vi "DO Block Config Pane.vi"(6 "_SubPanelMessages":refnum<notifier>, 9 "_myEmbeddedToFrameEvent":T7, 10 "_myEmbedded.Exit":refnum<user-event>, 11 "-Property Bundle":cluster{"Name":string, "Value":variant}[](array[cluster])) -> (1 "_Connection Informations":T3, 2 "_Scripter Input":T9)   [LabVIEW 2021]
doc: "Writes values to one or more digital output channels. Use this Express VI to write one or multiple samples for each channel at one time."
uses:
  <vilib>/myRIO/Common/Express VI Framework/xctls/myRIO Channel List/myRIO Channel List.xctl
  <vilib>/myRIO/Common/Express VI Framework/typedefs/Config Pane to Framework Ref.ctl
  <vilib>/myRIO/Common/Express VI Framework/typedefs/Data Validate Ref.ctl
  <vilib>/myRIO/Common/Express VI Framework/typedefs/Scripter Input.ctl
  <vilib>/myRIO/Common/Express VI Framework/typedefs/WireThrough Terminal Names.ctl
  <vilib>/myRIO/Common/Express VI Framework/typedefs/Instrument Driver Method Descriptor Array.ctl
  <vilib>/myRIO/Common/Express VI Framework/typedefs/Instrument Driver Method Descriptor.ctl
  <vilib>/myRIO/Common/Express VI Framework/typedefs/Sub Panel Messages.ctl
  <vilib>/myRIO/Common/Express VI Framework/typedefs/Connection Informations.ctl
  <vilib>/myRIO/Common/Instrument Driver Framework/Utilities/typedefs/Channel Types.ctl
  <vilib>/myRIO/Common/Express VI Framework/vis/Express VI Framework Strings Global.vi
panel:
  out "_learnMoreLatency":string="Gaps exist between sequential n samples generations. Learn more"
  out "_learnMoreFrequency":string="Detailed information about valid update rates for this Express VI. Learn more"
  in  "Wait Until Done?":bool caption="Wait until done?"
  in  "_Validate":bool
  in  "Sample Rate:":dbl=1.0 caption="Update rate:"
  in  "Sample Rate Unit":enum16{"kS/s", "MS/s"}(ring)
  in  "Name:":string="Digital output (n samples)" caption="Node name:"
  in  "Selected Channel List":T1[](xcontrol)=[{"Channel Name"=0, "Channel Alias"="", "Remove Channel"=FALSE, "Index"=0}]
  in  "_Default Alias String":string
  in  "_VI Default Name (Edit and make value default)":string="Digital output (n samples)"
  in  "_WireThrough Info (Edit and make value default)":T4={"WireThrough Top In"="DO (N Samples) Ref In", "WireThrough Bottom In"="error in (no error)", "WireThrough Top Out"="DO (N Samples) Ref Out", "WireThrough Bottom Out"="error out"}
  in  "_Template Array (Edit and make value default)":T5=[{"Function Name"="Smart Open", "VI Path"=path "<vilib>/myRIO/Instrument Drivers/Onboard IO/DO Block/vis", "Script"=TRUE, "Inputs"=[{"name"="Channel Names", "value"=variant, "Config Pane Only"=TRUE, "Build Array"=FALSE, "Bundle Cluster"=FALSE, "Show Term"=FALSE, "alias"=[], "Required Input"=FALSE}], "Outputs"=[], "VI Class"=enum."Open", "Controls Refs[]"=[], "Inline"=FALSE}, {"Function Name"="Open", "VI Path"=path "<vilib>/myRIO/Instrument Drivers/Onboard IO/DO Block/vis", "Script"=FALSE, "Inputs"=[{"name"="Channel Names", "value"=variant, "Config Pane Only"=TRUE, "Build Array"=FALSE, "Bundle Cluster"=FALSE, "Show Term"=FALSE, "alias"=[], "Required Input"=FALSE}], "Outputs"=[], "VI Class"=enum."Open", "Controls Refs[]"=[], "Inline"=FALSE}, {"Function Name"="Write", "VI Path"=path "<vilib>/myRIO/Instrument Drivers/Onboard IO/DO Block/vis", "Script"=TRUE, "Inputs"=[{"name"="Values", "value"=variant, "Config Pane Only"=FALSE, "Build Array"=TRUE, "Bundle Cluster"=FALSE, "Show Term"=TRUE, "alias"=[], "Required Input"=TRUE}, {"name"="Sample Rate [Hz]", "value"=variant, "Config Pane Only"=TRUE, "Build Array"=FALSE, "Bundle Cluster"=FALSE, "Show Term"=FALSE, "alias"=[], "Required Input"=FALSE}, {"name"="Wait Until Done?", "value"=variant, "Config Pane Only"=TRUE, "Build Array"=FALSE, "Bundle Cluster"=FALSE, "Show Term"=FALSE, "alias"=[], "Required Input"=FALSE}], "Outputs"=[], "VI Class"=enum."Data", "Controls Refs[]"=[], "Inline"=FALSE}, {"Function Name"="Close", "VI Path"=path "<vilib>/myRIO/Instrument Drivers/Onboard IO/DO Block/vis", "Script"=FALSE, "Inputs"=[], "Outputs"=[], "VI Class"=enum."Close", "Controls Refs[]"=[], "Inline"=FALSE}]
  in  "_Test Close":bool
  # "User Visible Area"
  # "NOTE: Tab Order has been set\nfor this Front Panel.\n1. Name: (string control)\n2. Add Channel (button)\n3. Selected Channel List (array)\n\nAll other controls are excluded \nfrom Tabbing order\n\nTo exlude a control from context\nhelp prefix its label text with a '-'"
  # "This Express VI waits until the write operation completes."
  # "Gap:"
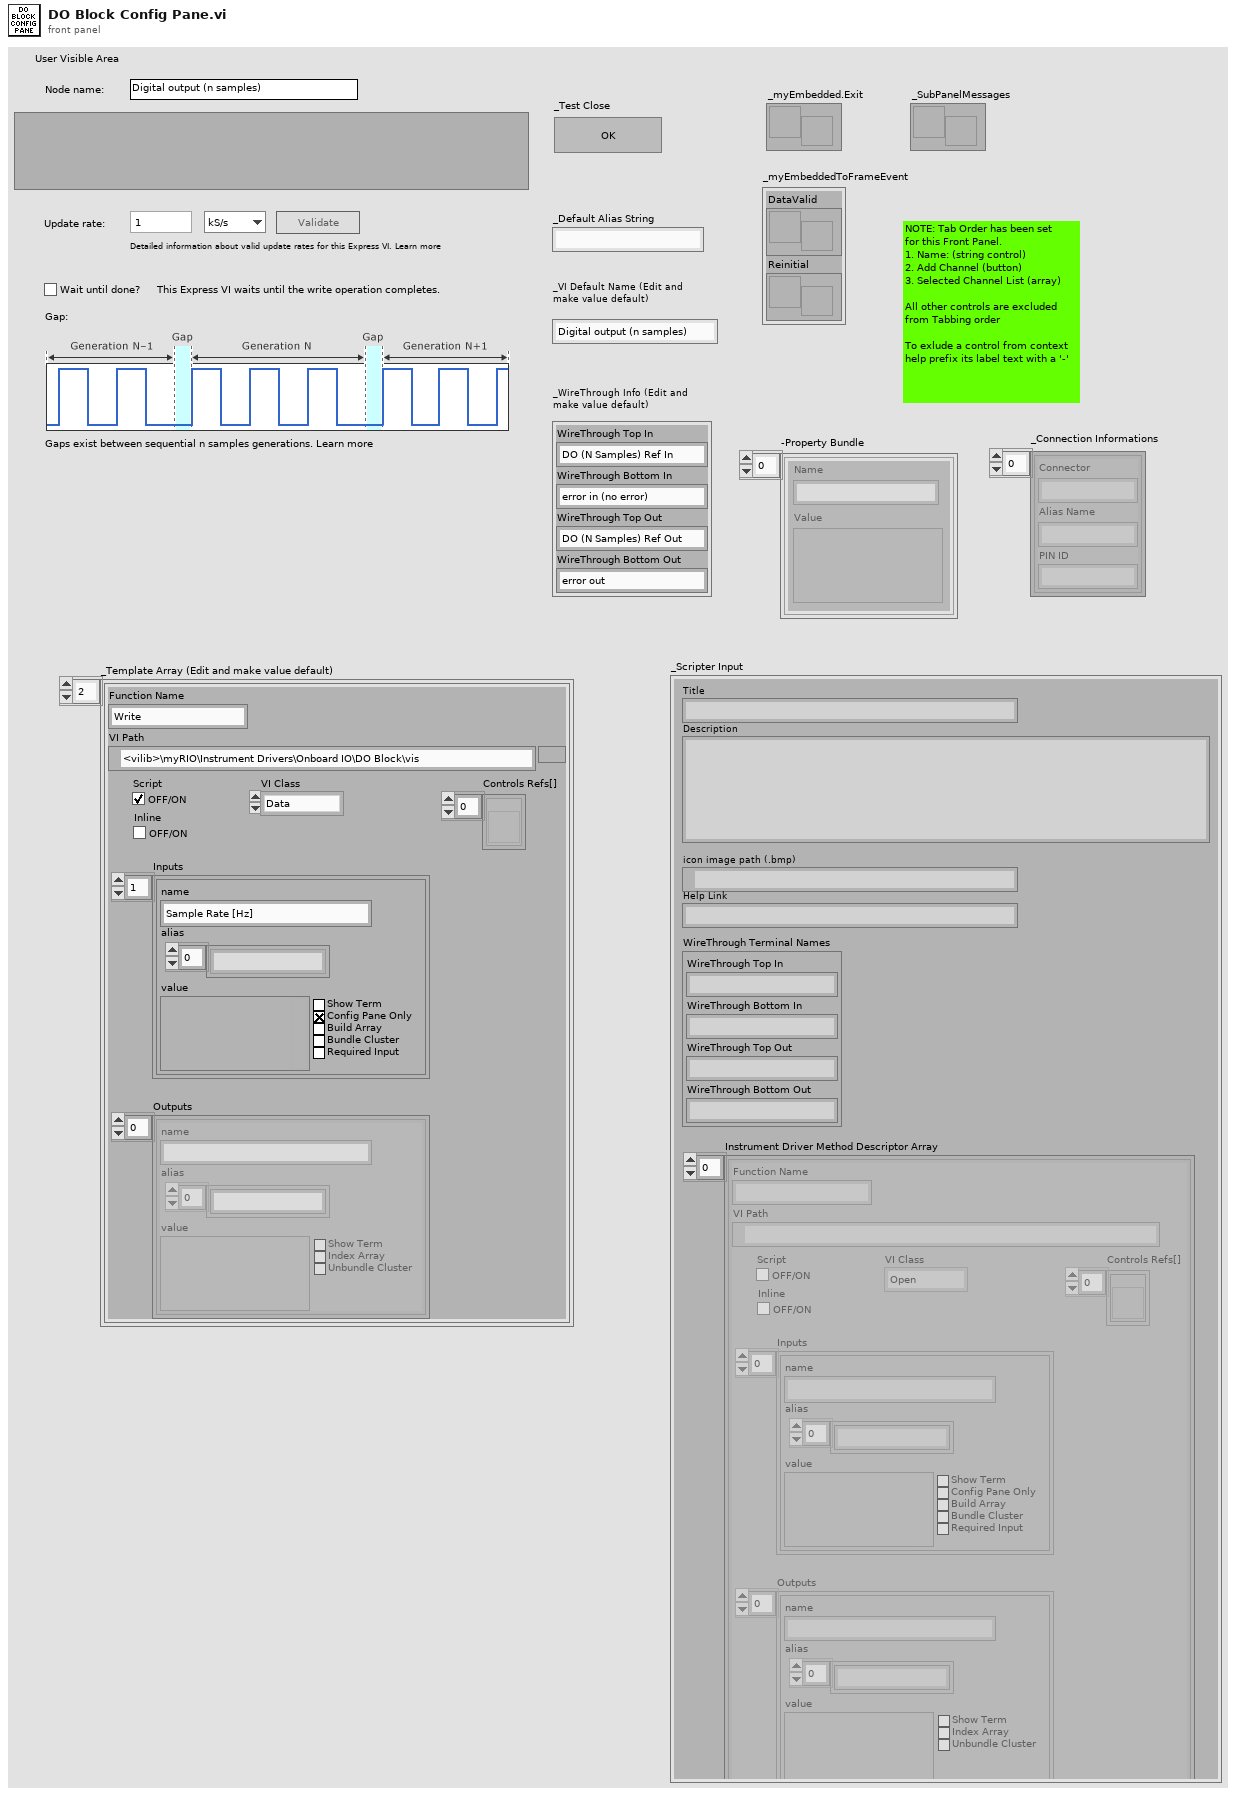
[diagram p1: front panel]
types:
  T1 = typedef "myRIO Channel List.xctl/Channel Data.ctl" = cluster{"Channel Name":u16, "Channel Alias":string, "Remove Channel":T2, "Index":i32}
  T2 = typedef "myRIO Channel List.xctl/Remove Channel.ctl" = bool
  T3 = typedef "Connection Informations.ctl" = cluster{"Connector":string, "Alias Name":string, "PIN ID":string}[]
  T4 = typedef "WireThrough Terminal Names.ctl" = cluster{"WireThrough Top In":string, "WireThrough Bottom In":string, "WireThrough Top Out":string, "WireThrough Bottom Out":string}
  T5 = typedef "Instrument Driver Method Descriptor Array.ctl" = T6[]
  T6 = typedef "Instrument Driver Method Descriptor.ctl" = cluster{"Function Name":string, "VI Path":path, "Script":bool, "Inputs":cluster{"name":string, "value":variant, "Config Pane Only":bool, "Build Array":bool, "Bundle Cluster":bool, "Show Term":bool, "alias":string[], "Required Input":bool}[], "Outputs":cluster{"name":string, "value":variant, "Show Term":bool, "Index Array":bool, "Unbundle Cluster":bool, "alias":string[]}[], "VI Class":enum16{"Open", "Configure", "Data", "Manage", "Close"}, "Controls Refs[]":refnum<vi>[], "Inline":bool}
  T7 = typedef "Config Pane to Framework Ref.ctl" = cluster{"DataValid":T8, "Reinitial":refnum<user-event>}
  T8 = typedef "Data Validate Ref.ctl" = refnum<user-event>
  T9 = typedef "Scripter Input.ctl" = cluster{"Title":string, "Description":string, "icon image path (.bmp)":path, "Help Link":string, "WireThrough Terminal Names":T4, "Instrument Driver Method Descriptor Array":T5}
  T10 = typedef "Channel Types.ctl" = enum32{"Unknown", "AI", "AO", "DIO - DI", "DIO", "DIO - DO", "I2C", "PWM", "Encoder", "SPI", "UART", "Accelerometer", "DIO - LED", "DIO - Button", "AI (N Samples)", "AudioIn (N Samples)", "AO (N Samples)", "AudioOut (N Samples)", "DI (N Samples)", "DO (N Samples)", "AI IRQ", "DI IRQ", "Timer IRQ", "RSL", "Relay", "CAN", "AI (Continuous)", "AO (Continuous)"}
  T11 = typedef "Channel Info.ctl" = cluster{"Channel Name":string, "Alias":string, "Used?":bool, "Not Support?":bool, "Property Bundle":cluster{"Name":string, "Value":variant}[]}
  T12 = typedef "Sub Panel Messages.ctl" = enum16{"Initialized"}
  T13 = enum8{"Enabled", "Disabled", "Disabled and Grayed Out"}
  T14 = cluster{"Connector":string, "Alias Name":string, "PIN ID":string}[]
  T15 = cluster{"name":string, "value":variant, "Config Pane Only":bool, "Build Array":bool, "Bundle Cluster":bool, "Show Term":bool, "alias":string[], "Required Input":bool}[]
  T16 = cluster{"name":string, "value":variant, "Config Pane Only":bool, "Build Array":bool, "Bundle Cluster":bool, "Show Term":bool, "alias":string[], "Required Input":bool}
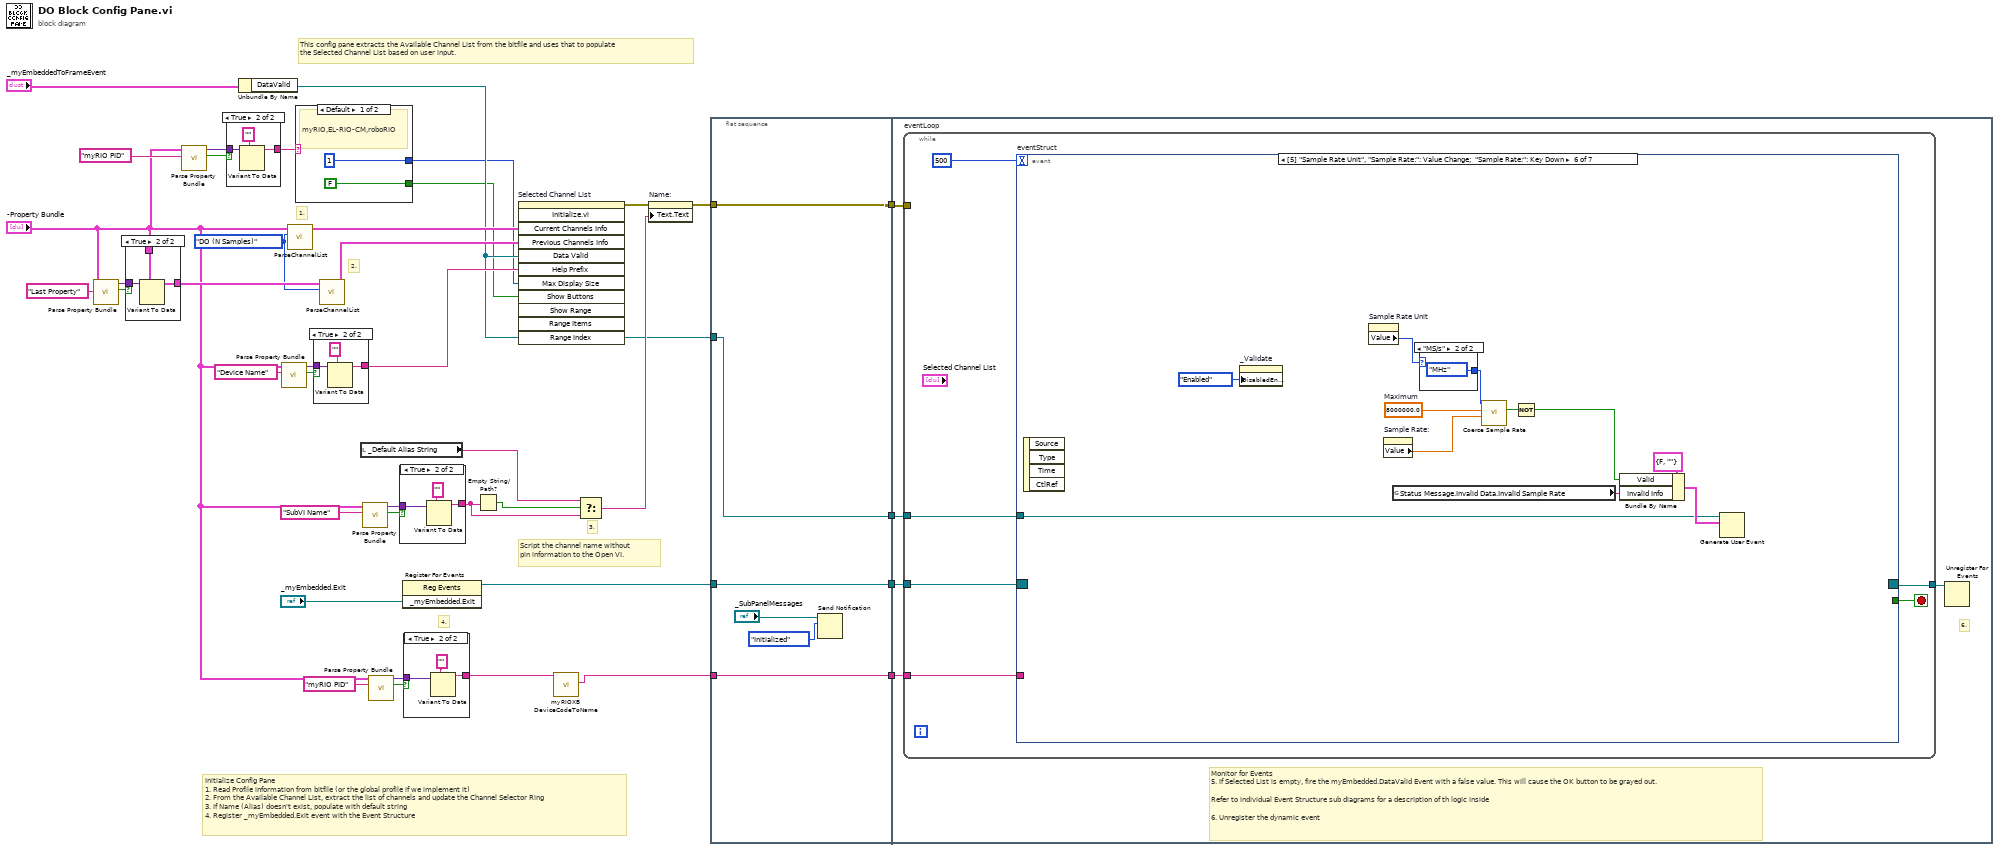
[diagram p0: block diagram]
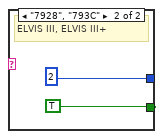
[diagram p2: hidden frame]
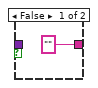
[diagram p3: hidden frame]
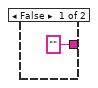
[diagram p4: hidden frame]
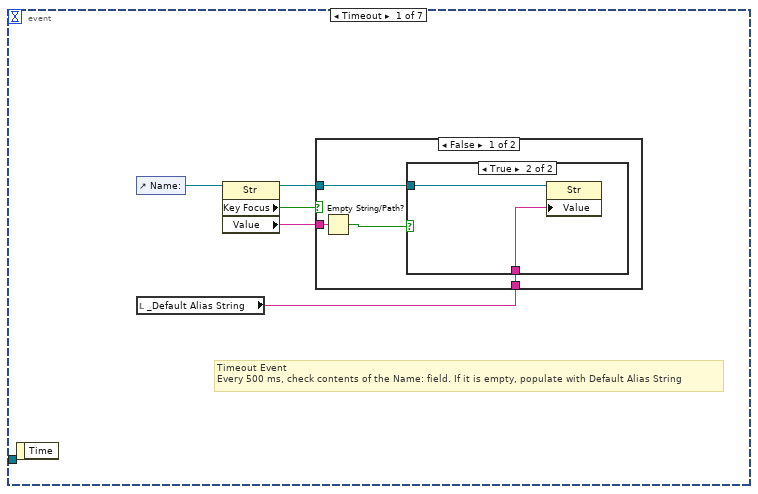
[diagram p5: hidden frame]
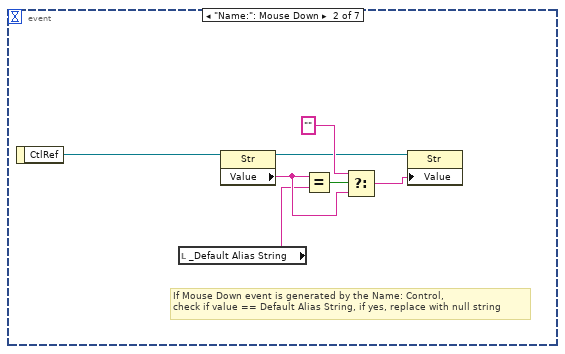
[diagram p8: hidden frame]
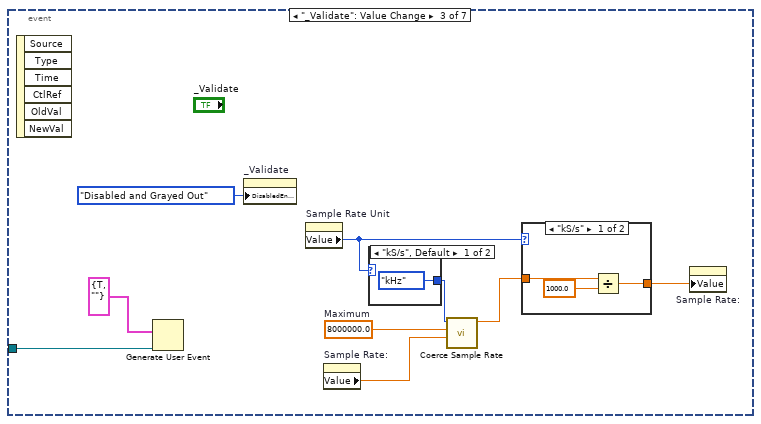
[diagram p9: hidden frame]
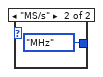
[diagram p10: hidden frame]
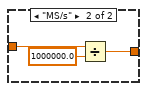
[diagram p11: hidden frame]
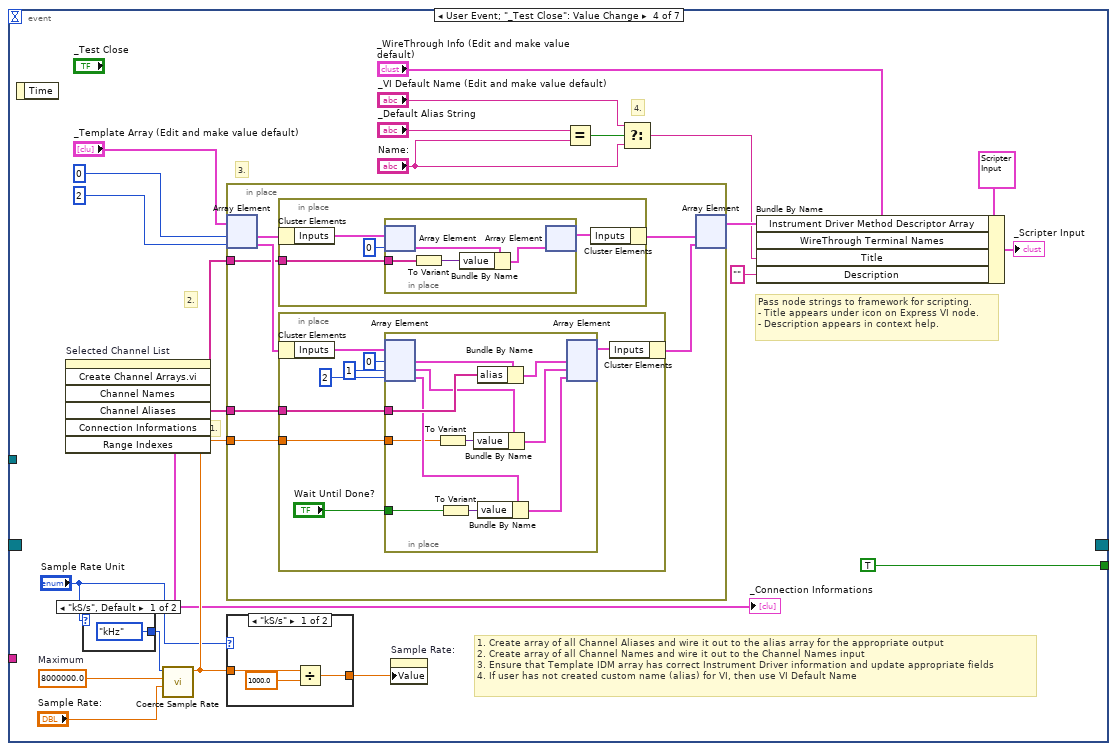
[diagram p12: hidden frame]
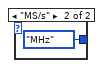
[diagram p13: hidden frame]
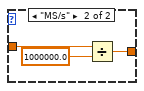
[diagram p14: hidden frame]
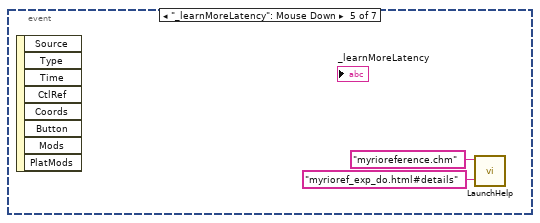
[diagram p15: hidden frame]
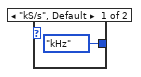
[diagram p16: hidden frame]
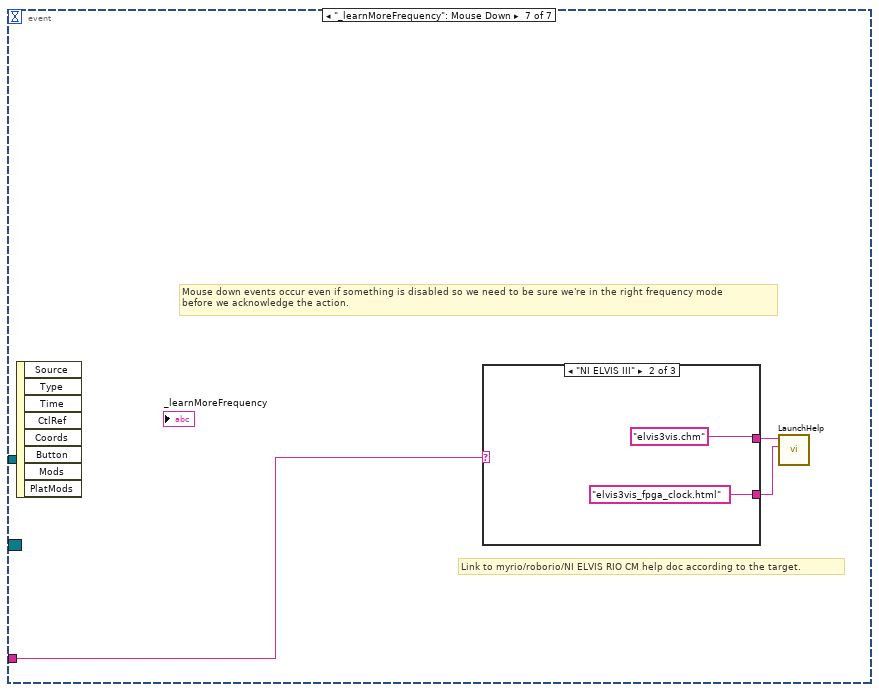
[diagram p17: hidden frame]
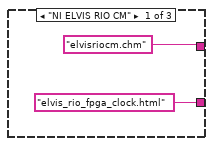
[diagram p18: hidden frame]
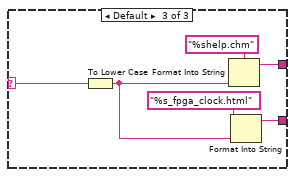
[diagram p19: hidden frame]
diagram:
  w24 = Channel_Types."DO (N Samples)" ("Channel to Read")
  # "2."
  # "1."
  # "Script the channel name without pin information to the Open VI."
  # "This config pane extracts the Available Channel List from the bitfile and uses that to populate\nthe Selected Channel List based on user input."
  # "4."
  # "3."
  # "Initialize Config Pane\n1. Read Profile information from bitfile (or the global profile if we implement it)\n2. From the Available Channel List, extract the list of channels and update the Channel Selector Ring\n3. If Name (Alias) doesn't exist, populate with default string\n4. Register _myEmbedded.Exit event with the Event Structure"
  n1 = call <vilib>:"Parse Property Bundle.vi"("Name"="Last Property", "Property Bundle"="-Property Bundle") -> ("Found?"=w26:bool, "Value"=w27:variant)  [unwired: 8 in]
  n2 = case shown="True" w26 {
    tunnel: w27 -> [_ w43]
    tunnel: [_ w42] -> w25
    tunnel: "-Property Bundle" -> [_ w41]
    frame False {
    }
    frame True {
      n3 = Variant To Data(type=w41, Variant=w43) -> (data=w42:cluster{"Name":string, "Value":variant}[])  [unwired: 1 in, 1 out]
    }
  }
  n4 = call <vilib>:"Parse Property Bundle.vi"("Name"="myRIO PID", "Property Bundle"="-Property Bundle") -> ("Found?"=w5:bool, "Value"=w6:variant)  [unwired: 8 in]
  n5 = case shown="True" w5 {
    tunnel: w6 -> [_ w47]
    tunnel: ["" ("Name") w46] -> w4
    frame False {
    }
    frame True {
      n6 = Variant To Data(type="" ("Name"), Variant=w47) -> (data=w46:string)  [unwired: 1 in, 1 out]
    }
  }
  n7 = Unbundle By Name("_myEmbeddedToFrameEvent") -> ("DataValid"=w15:T8)
  n8 = call <vilib>:"Parse Property Bundle.vi"("Name"="Device Name", "Property Bundle"="-Property Bundle") -> ("Found?"=w21:bool, "Value"=w20:variant)  [unwired: 8 in]
  n9 = call <vilib>:"ParseChannelList.vi"("Channel to Read"=w24, "_Property Bundle"="-Property Bundle") -> ("Channel List Out"=w29:T11[])  [unwired: 7 in, 2 out]
  n10 = case shown="Default" w4 {
    tunnel: [FALSE TRUE] -> w2
    tunnel: [1 ("Max Display Size") 2 ("Max Display Size")] -> w1
    frame Default {
      # "myRIO,EL-RIO-CM,roboRIO"
    }
    frame "7928", "793C" {
      # "ELVIS III, ELVIS III+"
    }
  }
  n11 = case shown="True" w21 {
    tunnel: w20 -> [_ w54]
    tunnel: [_ w53] -> w18
    frame False {
    }
    frame True {
      n12 = Variant To Data(type="", Variant=w54) -> (data=w53:string)  [unwired: 1 in, 1 out]
    }
  }
  n13 = call <vilib>:"ParseChannelList.vi"("Channel to Read"=w24, "_Property Bundle"=w25) -> ("Channel List Out"=w23:T11[])  [unwired: 7 in, 2 out]
  n14 = local read "_Default Alias String"() -> (w30:string)
  n15 = call <vilib>:"Parse Property Bundle.vi"("Name"="SubVI Name", "Property Bundle"="-Property Bundle") -> ("Found?"=w34:bool, "Value"=w33:variant)  [unwired: 8 in]
  n16 = call <vilib>:"Parse Property Bundle.vi"("Name"="myRIO PID", "Property Bundle"="-Property Bundle") -> ("Found?"=w11:bool, "Value"=w12:variant)  [unwired: 8 in]
  n17 = case shown="True" w34 {
    tunnel: w33 -> [_ w58]
    tunnel: ["" ("Name") w56] -> w32
    frame False {
    }
    frame True {
      n18 = Variant To Data(type="" ("Name"), Variant=w58) -> (data=w56:string)  [unwired: 1 in, 1 out]
    }
  }
  n19 = register-events("_myEmbedded.Exit") -> (reference out=w40:refnum<event-registration>)  [unwired: 2 in, 1 out]
  n20 = case shown="True" w11 {
    tunnel: w12 -> [_ w62]
    tunnel: ["" ("Name") w60] -> w9
    frame False {
    }
    frame True {
      n21 = Variant To Data(type="" ("Name"), Variant=w62) -> (data=w60:string)  [unwired: 1 in, 1 out]
    }
  }
  n22 = Empty String/Path?(string/path=w32) -> (empty?=w38:bool)
  n23 = invoke on="Selected Channel List" class="myRIO Channel List (strict)" method="Initialize.vi"("Current Channels Info"=w29, "Previous Channels Info"=w23, "Data Valid"=w15, "Help Prefix"=w18, "Max Display Size"=w1, "Show Buttons"=w2) -> (error out=w31:errorcluster)  [unwired: 6 in, 11 out]
  n24 = call <vilib>:"myRIOXB DeviceCodeToName.vi"("Device Code"=w9) -> ("Name"=w8:string)  [unwired: 10 in]
  n25 = Select(t=w30, s=w38, f=w32) -> (s? t:f=w37:string)
  n26 = property on="Name:" class="Str"(error in=w31, "Text.Text"=w37) -> (error out=w36:errorcluster)  [unwired: 1 in, 1 out]
  n27 = flat-sequence {
    tunnel: w36 -> [w67]
    tunnel: w40 -> [w68]
    tunnel: [w68] -> w17
    tunnel: [w67] -> w16
    tunnel: w15 -> [w64]
    tunnel: [w64] -> w14
    tunnel: w8 -> [w63]
    tunnel: [w63] -> w10
    tunnel: w17 -> [w73]
    tunnel: w16 -> [w71]
    tunnel: w14 -> [w70]
    tunnel: w10 -> [w69]
    frame #0 {
      n28 = Send Notification(notification=Sub_Panel_Messages."Initialized", notifier="_SubPanelMessages") -> ()  [unwired: 1 in, 2 out]
    }
    frame #1 {
      # "6."
      # "Monitor for Events\n5. If Selected List is empty, fire the myEmbedded.DataValid Event with a false value. This will cause the OK button to be grayed out.\n\nRefer to individual Event Structure sub diagrams for a description of th logic inside\n\n6. Unregister the dynamic event"
      n29 = while "eventLoop" {
        tunnel: w73 -> [w78]
        tunnel: [w77] -> w72
        tunnel: w71 -> [_]
        tunnel: w70 -> [w75]
        tunnel: w69 -> [w74]
        stop <- w79 stop-if-true
        n30 = event "eventStruct" shown="[5] \"Sample Rate Unit\", \"Sample Rate:\": Value Change;  \"Sample Rate:\": Key Down" {
          selector: w78 -> [_ _ _ _ _ _ _]
          dyn-events: [_ _ _ _ _ _ _] -> w77
          timeout: 500 -> [_ _ _ _ _ _ _]
          tunnel: [_ _ _ TRUE ("_Test Close") _ _ _] -> w79
          tunnel: w75 -> [_ _ w98 _ _ w184 _]
          tunnel: w74 -> [_ _ _ _ _ _ w195]
          event Timeout {
            # "Timeout Event\nEvery 500 ms, check contents of the Name: field. If it is empty, populate with Default Alias String"
            n31 = event-data() -> ()  [unwired: 1 in, 1 out]
            n32 = control-ref of="Name:"() -> (w82:refnum<vi>)
            n33 = local read "_Default Alias String"() -> (w80:string)
            n34 = property on="Property Node" class="Str"(reference=w82) -> (reference out=w81:refnum<vi>, "Key Focus"=w83:bool, "Value"=w84:string)  [unwired: 1 in, 1 out]
            n35 = case shown="False" w83 {
              tunnel: w84 -> [w88 _]
              tunnel: w81 -> [w86 _]
              tunnel: w80 -> [w85 _]
              frame False {
                n36 = Empty String/Path?(string/path=w88) -> (empty?=w87:bool)
                n37 = case shown="True" w87 {
                  tunnel: w86 -> [_ w90]
                  tunnel: w85 -> [_ w89]
                  frame False {
                  }
                  frame True {
                    n38 = property on="Property Node" class="Str"(reference=w90, "Value"=w89) -> ()  [unwired: 1 in, 2 out]
                  }
                }
              }
              frame True {
              }
            }
          }
          event "Name:": Mouse Down {
            # "If Mouse Down event is generated by the Name: Control,\ncheck if value == Default Alias String, if yes, replace with null string"
            n39 = event-data() -> ("CtlRef"=w97:refnum<vi>)  [unwired: 1 in]
            n40 = local read "_Default Alias String"() -> (w91:string)
            n41 = property class="Str"(reference=w97) -> (reference out=w93:refnum<vi>, "Value"=w92:string)  [unwired: 1 in, 1 out]
            n42 = Equal?(x=w92, y=w91) -> (x = y?=w96:bool)
            n43 = Select(t="", s=w96, f=w92) -> (s? t:f=w94:string)
            n44 = property class="Str"(reference=w93, "Value"=w94) -> ()  [unwired: 1 in, 2 out]
          }
          event "_Validate": Value Change {
            w106 = 8000000.0  # Maximum
            n45 = event-data() -> ()  [unwired: 1 in, 6 out]
            n46 = Generate User Event(user event=w98, event data cluster=cluster{"Valid":bool, "Invalid Info":string} {"Valid"=TRUE, "Invalid Info"=""} ("event data")) -> ()  [unwired: 2 in, 2 out]
            n47 = property on="_Validate" class="Bool"("DisabledEnum"=T13."Disabled and Grayed Out" ("Disabled")) -> ()  [unwired: 2 in, 2 out]
            n48 = property on="Sample Rate Unit" class="Enum (strict)"() -> ("Value"=w101:enum16{"kS/s", "MS/s"})  [unwired: 2 in, 2 out]
            n49 = property on="Sample Rate:" class="DigNum (strict)"() -> ("Value"=w104:dbl)  [unwired: 2 in, 2 out]
            n50 = case shown="\"kS/s\", Default" w101 {
              tunnel: [enum16{"Hz", "kHz", "MHz"}."kHz" ("Sample Rate Unit") enum16{"Hz", "kHz", "MHz"}."MHz" ("Sample Rate Unit")] -> w100
              frame "kS/s", Default {
              }
              frame "MS/s" {
              }
            }
            n51 = call <vilib>:"Coerce Sample Rate.vi"("Sample Rate:"=w104, "Maximum"=w106, "Sample Rate Unit"=w100) -> ("Actual Sample Rate (s)"=w105:dbl)  [unwired: 7 in, 1 out]
            n52 = case shown="\"kS/s\"" w101 {
              tunnel: w105 -> [w111 w113]
              tunnel: [w109 w112] -> w103
              frame "kS/s" {
                n53 = Divide(x=w111, y=1000.0) -> (x/y=w109:dbl)
              }
              frame "MS/s" {
                n54 = Divide(x=w113, y=1000000.0) -> (x/y=w112:dbl)
              }
            }
            n55 = property on="Sample Rate:" class="DigNum (strict)"("Value"=w103) -> ()  [unwired: 2 in, 2 out]
          }
          event User Event; "_Test Close": Value Change {
            w122 = 8000000.0  # Maximum
            # "1."
            # "2."
            # "1. Create array of all Channel Aliases and wire it out to the alias array for the appropriate output\n2. Create array of all Channel Names and wire it out to the Channel Names input\n3. Ensure that Template IDM array has correct Instrument Driver information and update appropriate fields\n4. If user has not created custom name (alias) for VI, then use VI Default Name"
            # "4."
            # "3."
            # "Pass node strings to framework for scripting.\n- Title appears under icon on Express VI node.\n- Description appears in context help."
            n56 = event-data() -> ()  [unwired: 1 in, 1 out]
            n57 = invoke on="Selected Channel List" class="myRIO Channel List (strict)" method="Create Channel Arrays.vi"() -> ("Channel Names"=w119:string[], "Channel Aliases"=w118:string[], "Connection Informations"=→"_Connection Informations":T14)  [unwired: 7 in, 4 out]
            n58 = case shown="\"kS/s\", Default" "Sample Rate Unit" {
              tunnel: [enum16{"Hz", "kHz", "MHz"}."kHz" ("Sample Rate Unit") enum16{"Hz", "kHz", "MHz"}."MHz" ("Sample Rate Unit")] -> w115
              frame "kS/s", Default {
              }
              frame "MS/s" {
              }
            }
            n59 = call <vilib>:"Coerce Sample Rate.vi"("Sample Rate:"="Sample Rate:", "Maximum"=w122, "Sample Rate Unit"=w115) -> ("Actual Sample Rate (s)"=w120:dbl)  [unwired: 7 in, 1 out]
            n60 = in-place {
              in-place-border: w119 -> [w148]
              in-place-border: w118 -> [w147]
              in-place-border: w120 -> [w146]
              n61 = in-place-array #1("_Template Array (Edit and make value default)", 0, 2) -> (w152:T6, w150:T6)
              n62 = in-place {
                in-place-border: w148 -> [w174]
                n63 = in-place-cluster #2(w152) -> ("Inputs"=w175:T15)
                n64 = in-place {
                  in-place-border: w174 -> [w176]
                  n65 = in-place-array #3(w175, 0) -> (w179:T16)
                  n66 = To Variant(anything=w176) -> (Variant=w177:variant)
                  n67 = Bundle By Name(cluster=w179, "value"=w177) -> (w178:T16)
                  n68 = in-place-array #3(w178) -> (w173:T15)  [unwired: 1 out]
                }
                n69 = in-place-cluster #2("Inputs"=w173) -> (w151:T6)
              }
              n70 = in-place {
                in-place-border: w147 -> [w159]
                in-place-border: w146 -> [w154]
                n71 = in-place-cluster #4(w150) -> ("Inputs"=w160:T15)
                n72 = in-place {
                  in-place-border: w159 -> [w169]
                  in-place-border: w154 -> [w164]
                  in-place-border: "Wait Until Done?" -> [w163]
                  n73 = in-place-array #5(w160, 0, 1, 2) -> (w171:T16, w168:T16, w167:T16)
                  n74 = To Variant(anything=w164) -> (Variant=w166:variant)
                  n75 = To Variant(anything=w163) -> (Variant=w165:variant)
                  n76 = Bundle By Name(cluster=w168, "value"=w166) -> (w162:T16)
                  n77 = Bundle By Name(cluster=w171, "alias"=w169) -> (w170:T16)
                  n78 = Bundle By Name(cluster=w167, "value"=w165) -> (w161:T16)
                  n79 = in-place-array #5(w170, w162, w161) -> (w158:T15)  [unwired: 3 out]
                }
                n80 = in-place-cluster #4("Inputs"=w158) -> (w149:T6)
              }
              n81 = in-place-array #1(w151, w149) -> (w135:T5)  [unwired: 2 out]
            }
            n82 = case shown="\"kS/s\"" "Sample Rate Unit" {
              tunnel: w120 -> [w142 w144]
              tunnel: [w140 w143] -> w123
              frame "kS/s" {
                n83 = Divide(x=w142, y=1000.0) -> (x/y=w140:dbl)
              }
              frame "MS/s" {
                n84 = Divide(x=w144, y=1000000.0) -> (x/y=w143:dbl)
              }
            }
            n85 = property on="Sample Rate:" class="DigNum (strict)"("Value"=w123) -> ()  [unwired: 2 in, 2 out]
            n86 = Equal?(x="_Default Alias String", y="Name:") -> (x = y?=w127:bool)
            n87 = Select(t="_VI Default Name (Edit and make value default)", s=w127, f="Name:") -> (s? t:f=w125:string)
            n88 = Bundle By Name(cluster=T9 {"Title"="", "Description"="", "icon image path (.bmp)"=path "", "Help Link"="", "WireThrough Terminal Names"={"WireThrough Top In"="", "WireThrough Bottom In"="", "WireThrough Top Out"="", "WireThrough Bottom Out"=""}, "Instrument Driver Method Descriptor Array"=[]} ("Scripter Input"), "Instrument Driver Method Descriptor Array"=w135, "WireThrough Terminal Names"="_WireThrough Info (Edit and make value default)", "Title"=w125, "Description"="" ("Title")) -> (→"_Scripter Input":T9)
          }
          event "_learnMoreLatency": Mouse Down {
            n89 = event-data() -> ()  [unwired: 1 in, 8 out]
            n90 = call <vilib>:"LaunchHelp.vi"("Help Topic"="myrioref_exp_do.html#details", "Help File"="myrioreference.chm") -> ()  [unwired: 10 in]
          }
          event "Sample Rate Unit", "Sample Rate:": Value Change; "Sample Rate:": Key Down {
            w191 = 8000000.0  # Maximum
            n91 = event-data() -> ()  [unwired: 1 in, 4 out]
            n92 = property on="_Validate" class="Bool"("DisabledEnum"=T13."Enabled" ("Disabled")) -> ()  [unwired: 2 in, 2 out]
            n93 = property on="Sample Rate Unit" class="Enum (strict)"() -> ("Value"=w189:enum16{"kS/s", "MS/s"})  [unwired: 2 in, 2 out]
            n94 = property on="Sample Rate:" class="DigNum (strict)"() -> ("Value"=w190:dbl)  [unwired: 2 in, 2 out]
            n95 = global read "Express VI Framework Strings Global.vi" "Status Message.Invalid Data.Invalid Sample Rate"() -> (w185:string)
            n96 = case shown="\"MS/s\"" w189 {
              tunnel: [enum16{"Hz", "kHz", "MHz"}."kHz" ("Sample Rate Unit") enum16{"Hz", "kHz", "MHz"}."MHz" ("Sample Rate Unit")] -> w188
              frame "kS/s", Default {
              }
              frame "MS/s" {
              }
            }
            n97 = call <vilib>:"Coerce Sample Rate.vi"("Sample Rate:"=w190, "Maximum"=w191, "Sample Rate Unit"=w188) -> ("Coercion needed?"=w183:bool)  [unwired: 7 in, 1 out]
            n98 = Not(x=w183) -> (.not. x?=w182:bool)
            n99 = Bundle By Name(cluster=cluster{"Valid":bool, "Invalid Info":string} {"Valid"=FALSE, "Invalid Info"=""} ("event data"), "Valid"=w182, "Invalid Info"=w185) -> (w186:cluster{"Valid":bool, "Invalid Info":string})
            n100 = Generate User Event(user event=w184, event data cluster=w186) -> ()  [unwired: 2 in, 2 out]
          }
          event "_learnMoreFrequency": Mouse Down {
            # "Link to myrio/roborio/NI ELVIS RIO CM help doc according to the target."
            # "Mouse down events occur even if something is disabled so we need to be sure we're in the right frequency mode\nbefore we acknowledge the action."
            n101 = event-data() -> ()  [unwired: 1 in, 8 out]
            n102 = case shown="\"NI ELVIS III\"" w195 {
              selector: w195 -> [_ _ w202]
              tunnel: ["elvisriocm.chm" ("Help File") "elvis3vis.chm" ("Help File") w204] -> w197
              tunnel: ["elvis_rio_fpga_clock.html" ("Help Topic") "elvis3vis_fpga_clock.html" ("Help Topic") w203] -> w196
              frame "NI ELVIS RIO CM" {
              }
              frame "NI ELVIS III" {
              }
              frame Default {
                n103 = To Lower Case(string=w202) -> (all lower case string=w206:string)
                n104 = Format Into String(format string="%shelp.chm" ("Help File"), w206) -> (resulting string=w204:string)  [unwired: 2 in, 1 out]
                n105 = Format Into String(format string="%s_fpga_clock.html" ("Help Topic"), w206) -> (resulting string=w203:string)  [unwired: 2 in, 1 out]
              }
            }
            n106 = call <vilib>:"LaunchHelp.vi"("Help Topic"=w196, "Help File"=w197) -> ()  [unwired: 10 in]
          }
        }
      }
      n107 = Unregister For Events(event registration refnum=w72) -> ()  [unwired: 1 in, 1 out]
    }
  }
